vi "Read IMU (Consumer).vi"() -> (0 "Thigh Angle [rad]":dbl, 1 "Yaw Angle [rad]":dbl, 2 "Pitch Angle [rad]":dbl, 3 "Roll Angle [rad]":dbl)   [LabVIEW 2018]
uses:
  <vilib>/Analysis/3filter.llb/Filter Passband Type.ctl
  <vilib>/ptbypt/NI_PtbyPt.lvlib
  <vilib>/Analysis/NI_AALBase.lvlib
panel:
  out "Corrected Hex":string
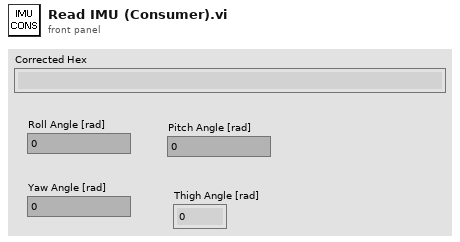
[diagram p1: front panel]
types:
  T1 = typedef "NI_AALBase.lvlib/Filter Passband Type.ctl" = enum32{"Lowpass", "Highpass", "Bandpass", "Bandstop"}
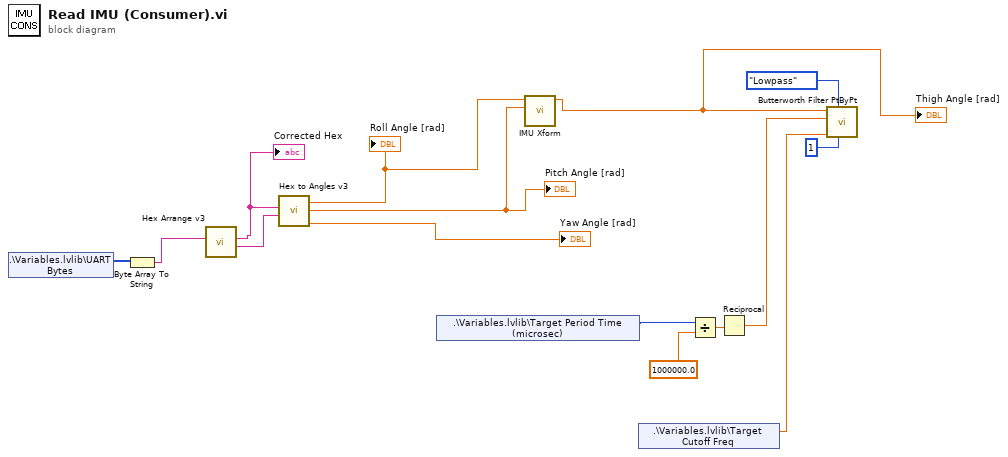
[diagram p0: block diagram]
diagram:
  n1 = shared-variable ".\\Variables.lvlib\\UART Bytes"() -> (w15:u8[])  [unwired: 1 in, 1 out]
  n2 = Byte Array To String(unsigned byte array=w15) -> (string=w14:string)
  n3 = call "Hex Arrange v3.vi"("Hex from UART"=w14) -> ("after substring"=w11:string, "Corrected Hex"=w13:string)  [unwired: 9 in]
  "Corrected Hex" <- w13
  n4 = call "Hex to Angles v3.vi"("Hex after Headers"=w11, "Hex from UART"=w13) -> ("Yaw Angle [rad]"=→"Yaw Angle [rad]":dbl, "Pitch Angle [rad]"=w2:dbl, "Roll Angle [rad]"=w3:dbl)  [unwired: 7 in]
  "Roll Angle [rad]" <- w3
  "Pitch Angle [rad]" <- w2
  n5 = shared-variable ".\\Variables.lvlib\\Target Period Time (microsec)"() -> (w8:u16)  [unwired: 1 in, 1 out]
  n6 = call "IMU Xform.vi"("Pitch"=w2, "Roll"=w3) -> ("Thigh Angle"=w1:dbl)  [unwired: 9 in]
  "Thigh Angle [rad]" <- w1
  n7 = shared-variable ".\\Variables.lvlib\\Target Cutoff Freq"() -> (w6:dbl)  [unwired: 1 in, 1 out]
  n8 = Divide(x=w8, y=1000000.0) -> (x/y=w10:dbl)
  n9 = Reciprocal(x=w10) -> (1/x=w7:dbl)
  n10 = call <vilib>:"Butterworth Filter PtByPt.vi"("order"=1, "filter type"=Filter_Passband_Type."Lowpass", "low cutoff freq: fl"=w6, "sampling freq: fs"=w7, "x"=w1) -> ()  [unwired: 4 in, 2 out]
